vi "Align Needle Dialog.vi"(7 "Console Log in":refnum<class "Console Log.lvclass">, 8 "error in":errorcluster, 11 "Potting Procedure in":refnum<class "Potting Procedure.lvclass">) -> (0 "error out":errorcluster, 2 "Canceled":bool, 3 "Potting Procedure out":refnum<class "Potting Procedure.lvclass">, 5 "Console Log out":refnum<class "Console Log.lvclass">)   [LabVIEW 2011]
uses:
  Procedure Classes/Potting Procedure/Potting Procedure.lvclass
  UI Classes/Console Log/Console Log.lvclass
  Shared Components/Gantry Class/Gantry Class.lvclass
  Shared Components/Vec3d Class/Vec3d Class.lvclass
  Shared Components/WorkTable Class/WorkTable Class.lvclass
panel:
  out "Offset(mm)":cluster{"X":dbl, "Y":dbl, "Z":dbl}
  in  "Camera Selection":enum32{"Radio Selection 1", "Radio Selection 2"}(radio)
  out "preview":T1(plugin-control)
  in  "OK Button":bool
  in  "Cancel Button":bool
  # "Use the MPG  hand control to\nmove the needle tip to the center\nof the image in both X and Y"
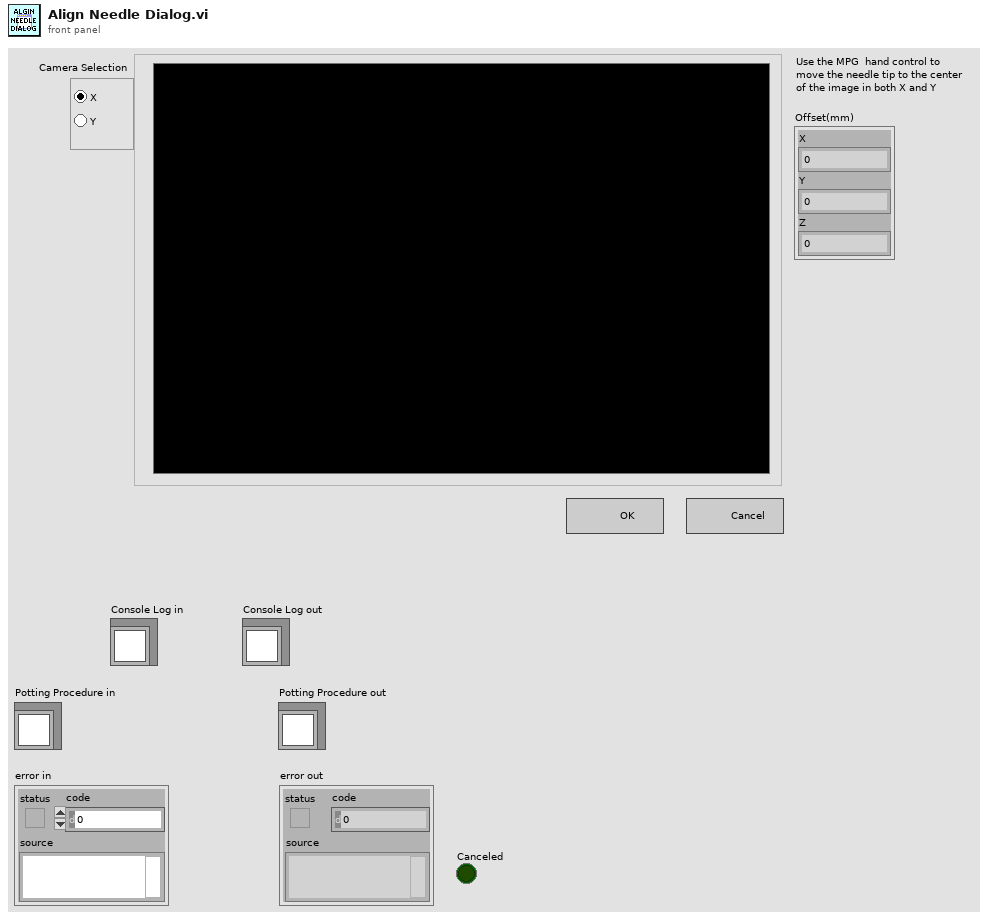
[diagram p1: front panel]
types:
  T1 = typedef "IMAQ Image.ctl" = refnum<image>
  T2 = enum8{"Enabled", "Disabled", "Disabled and Grayed Out"}
  T3 = typedef "Physical Image.ctl" = cluster{"Image Position":refnum<class "Vec3d Class.lvclass">, "Image Reference":T1, "Field of View":cluster{"x(mm)":dbl, "y(mm)":dbl}}
  T4 = typedef "Worktable_Syringe.ctl" = cluster{"Syringe Holder":enum16{"Empty", "Populated", "Calibrated"}, "Mixing Time":timestamp, "Tip Offset":refnum<class "Vec3d Class.lvclass">}
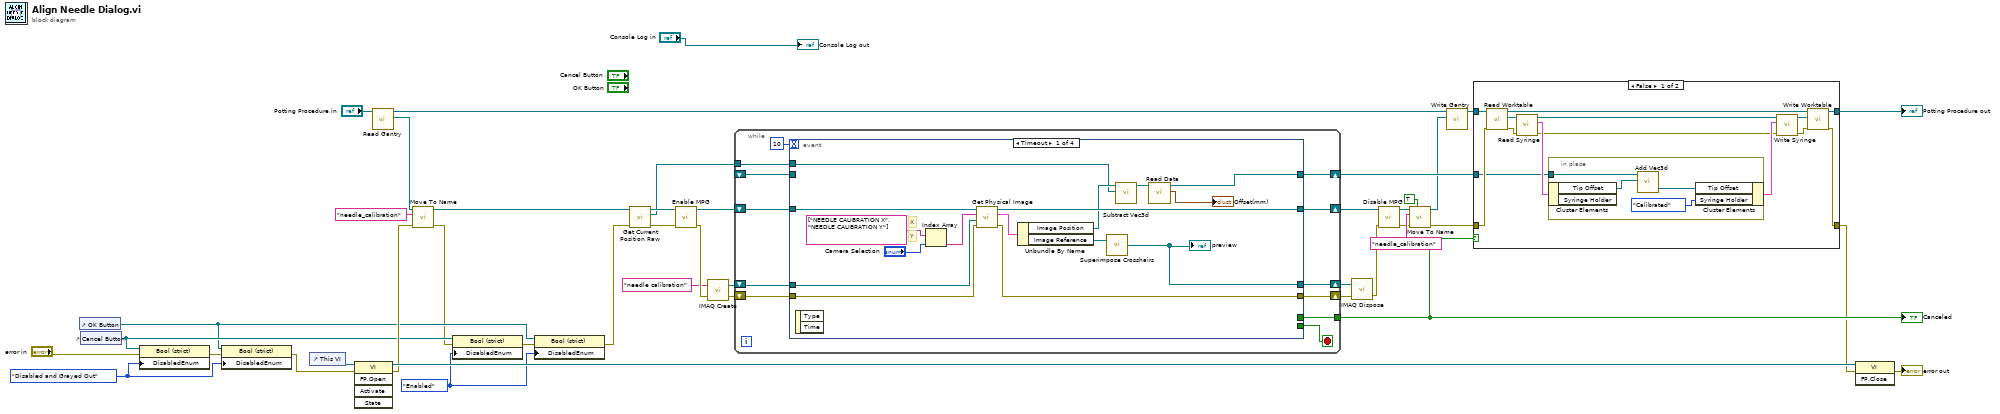
[diagram p0: block diagram]
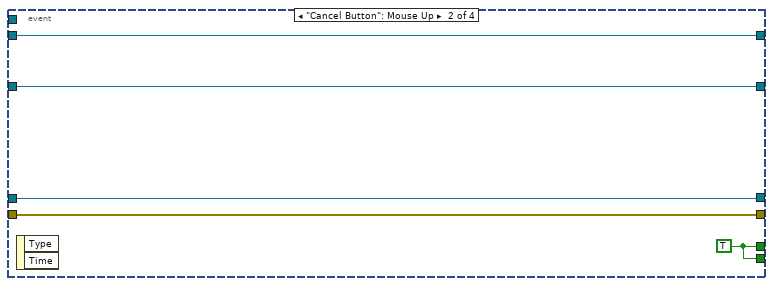
[diagram p3: hidden frame]
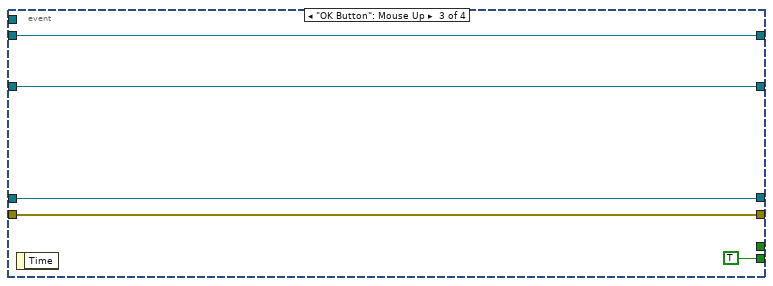
[diagram p4: hidden frame]
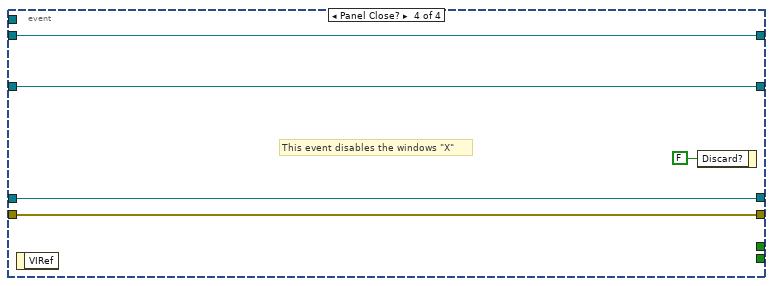
[diagram p5: hidden frame]
diagram:
  w6 = T2."Enabled" ("Disabled")
  w7 = T2."Disabled and Grayed Out" ("Disabled")
  n1 = control-ref of="OK Button"() -> (w8:refnum<vi>)
  n2 = control-ref of="Cancel Button"() -> (w9:refnum<vi>)
  n3 = property class="Bool (strict)"(reference=w9, error in="error in", "DisabledEnum"=w7) -> (error out=w11:errorcluster)  [unwired: 1 out]
  n4 = property class="Bool (strict)"(reference=w8, error in=w11, "DisabledEnum"=w7) -> (error out=w5:errorcluster)  [unwired: 1 out]
  n5 = control-ref of="This VI"() -> (w43:refnum<vi>)
  n6 = invoke class="VI" method="FP.Open"(reference=w43, error in=w5) -> (reference out=w42:refnum<vi>, error out=w37:errorcluster)  [unwired: 3 in, 3 out]
  n7 = call-dynamic "Read Gantry.vi"("Potting Procedure in"="Potting Procedure in") -> ("Gantry"=w39:refnum<class "Gantry Class.lvclass">, "Potting Procedure out"=w22:refnum<class "Potting Procedure.lvclass">)  [unwired: 8 in, 1 out]
  n8 = call-dynamic "Move To Name.vi"("error in"=w37, "Destination Name"="needle_calibration", "Gantry in"=w39) -> ("error out"=w3:errorcluster, "Gantry out"=w36:refnum<class "Gantry Class.lvclass">)  [unwired: 7 in]
  n9 = property class="Bool (strict)"(reference=w9, error in=w3, "DisabledEnum"=w6) -> (error out=w10:errorcluster)  [unwired: 1 out]
  n10 = property class="Bool (strict)"(reference=w8, error in=w10, "DisabledEnum"=w6) -> (error out=w2:errorcluster)  [unwired: 1 out]
  n11 = call-dynamic "Get Current Position Raw.vi"("error in (no error)"=w2, "Gantry Class in"=w36) -> ("error out"=w32:errorcluster, "Vec3d Class out"=w25:refnum<class "Vec3d Class.lvclass">, "Gantry Class out"=w35:refnum<class "Gantry Class.lvclass">)  [unwired: 7 in]
  n12 = call-dynamic "Enable MPG.vi"("error in (no error)"=w32, "Gantry Class in"=w35) -> ("error out"=w31:errorcluster, "Gantry Class out"=w34:refnum<class "Gantry Class.lvclass">)  [unwired: 8 in]
  n13 = call "IMAQ Create"("Image Name"="needle calibration", "error in (no error)"=w31) -> ("New Image"=w28:T1, "error out"=w29:errorcluster)  [unwired: 3 in]
  n14 = while {
    tunnel: [w51] -> w23
    shift-right: [w49] -> w33
    shift-left: w34 -> [w50]
    shift-right: [w53] -> w27
    shift-left: w29 -> [w52]
    shift-right: [w47] -> w26
    shift-left: w28 -> [w48]
    tunnel: w25 -> [w46]
    shift-right: [w45] -> w20
    shift-left: _ -> [w44]
    stop <- w54 stop-if-true
    n15 = event shown="[0] Timeout" {
      selector: _ -> [_ _ _ _]
      dyn-events: _ -> [_ _ _ _]
      timeout: 10 -> [_ _ _ _]
      tunnel: [_ w75 TRUE _] -> w54
      tunnel: [w62 w76 w81 w85] -> w53
      tunnel: w52 -> [w63 w76 w81 w85]
      tunnel: [_ w75 _ _] -> w51
      tunnel: w50 -> [w69 w73 w78 w83]
      tunnel: [w67 w73 w78 w83] -> w49
      tunnel: w48 -> [w64 w72 w77 w82]
      tunnel: [w61 w72 w77 w82] -> w47
      tunnel: w46 -> [w56 _ _ _]
      tunnel: [w58 w74 w79 w84] -> w45
      tunnel: w44 -> [_ w74 w79 w84]
      event Timeout {
        # "Y"
        # "X"
        n16 = event-data() -> ()  [unwired: 1 in, 2 out]
        n17 = Index Array(array=string[] ["NEEDLE CALIBRATION X", "NEEDLE CALIBRATION Y"], index="Camera Selection") -> (element=w68:string)
        n18 = call-dynamic "Get Physical Image.vi"("error in"=w63, "Image In"=w64, "Camera Name"=w68, "Gantry in"=w69) -> ("error out"=w62:errorcluster, "Physical Image"=w66:T3, "Gantry out"=w67:refnum<class "Gantry Class.lvclass">)  [unwired: 5 in]
        n19 = Unbundle By Name(w66) -> ("Image Position"=w60:refnum<class "Vec3d Class.lvclass">, "Image Reference"=w65:T1)
        n20 = call "Superimpose Crosshairs.vi"("Refnum in"=w65) -> ("Refnum out"=w61:T1)  [unwired: 1 in]
        "preview" <- w61
        n21 = call "Subtract Vec3d.vi"("Vec3d in 2"=w56, "Vec3d in 1"=w60) -> ("Vec3d Class out"=w59:refnum<class "Vec3d Class.lvclass">)  [unwired: 8 in, 1 out]
        n22 = call-dynamic "Read Data.vi"("Vec3d Class in"=w59) -> ("Data"=→"Offset(mm)":cluster{"X":dbl, "Y":dbl, "Z":dbl}, "Vec3d Class out"=w58:refnum<class "Vec3d Class.lvclass">)  [unwired: 8 in, 1 out]
      }
      event "Cancel Button": Mouse Up {
        w75 = TRUE
        n23 = event-data() -> ()  [unwired: 1 in, 2 out]
      }
      event "OK Button": Mouse Up {
        n24 = event-data() -> ()  [unwired: 1 in, 1 out]
      }
      event Panel Close? {
        # "This event disables the windows \"X\""
        n25 = event-data() -> ()  [unwired: 1 in, 1 out]
        n26 = event-data("Discard?"=FALSE) -> ()  [unwired: 1 in, 1 out]
      }
    }
  }
  "Canceled" <- w23
  n27 = call "IMAQ Dispose"("Image"=w26, "error in (no error)"=w27) -> ("error out"=w24:errorcluster)  [unwired: 4 in]
  n28 = call-dynamic "Disable MPG.vi"("error in"=w24, "Gantry in"=w33) -> ("error out"=w16:errorcluster, "Gantry out"=w15:refnum<class "Gantry Class.lvclass">)  [unwired: 8 in]
  n29 = call-dynamic "Move To Name.vi"("Move if Same"=TRUE, "error in"=w16, "Destination Name"="needle_calibration", "Gantry in"=w15) -> ("error out"=w12:errorcluster, "Gantry out"=w13:refnum<class "Gantry Class.lvclass">)  [unwired: 6 in]
  n30 = call-dynamic "Write Gantry.vi"("Gantry"=w13, "Potting Procedure in"=w22) -> ("Potting Procedure out"=w21:refnum<class "Potting Procedure.lvclass">)  [unwired: 8 in, 1 out]
  n31 = case shown="False" w23 {
    tunnel: w12 -> [w91 w105]
    tunnel: w21 -> [w96 w106]
    tunnel: [w92 w106] -> w19
    tunnel: w20 -> [w89 _]
    tunnel: [w87 w105] -> w18
    frame False {
      n32 = call-dynamic "Read Worktable.vi"("error in"=w91, "Potting Procedure in"=w96) -> ("error out"=w90:errorcluster, "WorkTable out"=w95:refnum<class "WorkTable Class.lvclass">, "Potting Procedure out"=w93:refnum<class "Potting Procedure.lvclass">)  [unwired: 7 in]
      n33 = call "Read Syringe.vi"("error in"=w90, "WorkTable in"=w95) -> ("error out"=w97:errorcluster, "Syringe"=w100:T4, "WorkTable out"=w98:refnum<class "WorkTable Class.lvclass">)  [unwired: 7 in]
      n34 = in-place {
        in-place-border: w89 -> [w101]
        n35 = in-place-cluster #1(w100) -> ("Tip Offset"=w102:refnum<class "Vec3d Class.lvclass">)  [unwired: 1 out]
        n36 = call-dynamic "Add Vec3d.vi"(10:"Vec3d Class in"=w102, 11:"Vec3d Class in"=w101) -> ("Vec3d Class out"=w103:refnum<class "Vec3d Class.lvclass">)  [unwired: 8 in, 1 out]
        n37 = in-place-cluster #1("Tip Offset"=w103, "Syringe Holder"=enum16{"Empty", "Populated", "Calibrated"}."Calibrated") -> (w99:T4)
      }
      n38 = call-dynamic "Write Syringe.vi"("error in (no error)"=w97, "Syringe"=w99, "WorkTable Class in"=w98) -> ("error out"=w88:errorcluster, "WorkTable Class out"=w94:refnum<class "WorkTable Class.lvclass">)  [unwired: 7 in]
      n39 = call-dynamic "Write Worktable.vi"("error in"=w88, "WorkTable in"=w94, "Potting Procedure in"=w93) -> ("error out"=w87:errorcluster, "Potting Procedure out"=w92:refnum<class "Potting Procedure.lvclass">)  [unwired: 7 in]
    }
    frame True {
    }
  }
  "Potting Procedure out" <- w19
  n40 = invoke class="VI" method="FP.Close"(reference=w42, error in=w18) -> (error out=→"error out":errorcluster)  [unwired: 1 in, 2 out]
  "Console Log out" <- "Console Log in"
